vi "Item Selection Demo.vi"() -> ()   [LabVIEW 2020]
doc: "This is a Demo VI used to demonstrate how the listbox and tree selection VIs work. Run the VI and then select items by clicking the symbols of the controls. Use Shift to select multiple items, and right click the control to use other options.\n-------------\nBrian Hoover (hooovahh)"
uses:
  Selection Global Method.ctl
panel:
  out "Tree Selection":string[](array[string])
  in  "Tree":string(tree)
  out "MCLB Selection":string[](array[string])
  out "SCLB Selection":string[](array[string])
  in  "Multicolumn Listbox":i32(listbox)=-1
  in  "Listbox":i32(listbox)=-1
  # "1) Run This VI\n2) Click the checkboxes to select and unselect items.\n3) Shift can be held to change the selection of multiple items\n4) Right click the control to change the selection.\n5) Disabled items cannot be changed."
  # "Tree controls are supported with selection and deselection of parents affecting the children.  Deselecting and selecting children also will change the icon of the parent."
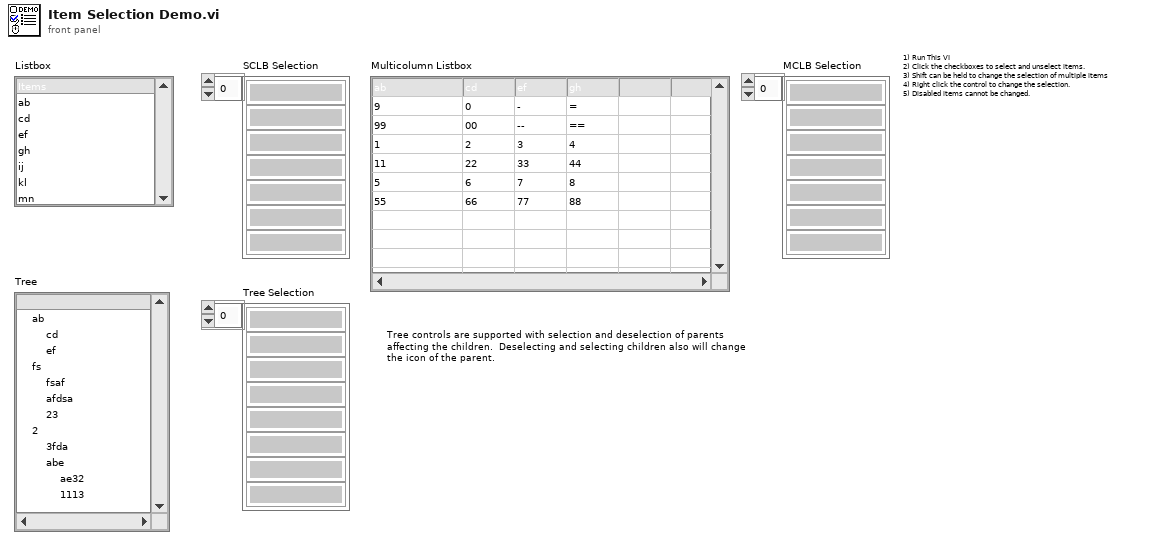
[diagram p1: front panel]
types:
  T1 = typedef "Selection Global Method.ctl" = enum16{"Read Selection", "Force Selection", "Mouse Down Event", "Select All", "Select None", "Invert Selection", "Read Selection and Tags"}
  T2 = typedef "LVPoint32TypeDef.ctl" = cluster{"Horizontal":i32, "Vertical":i32}
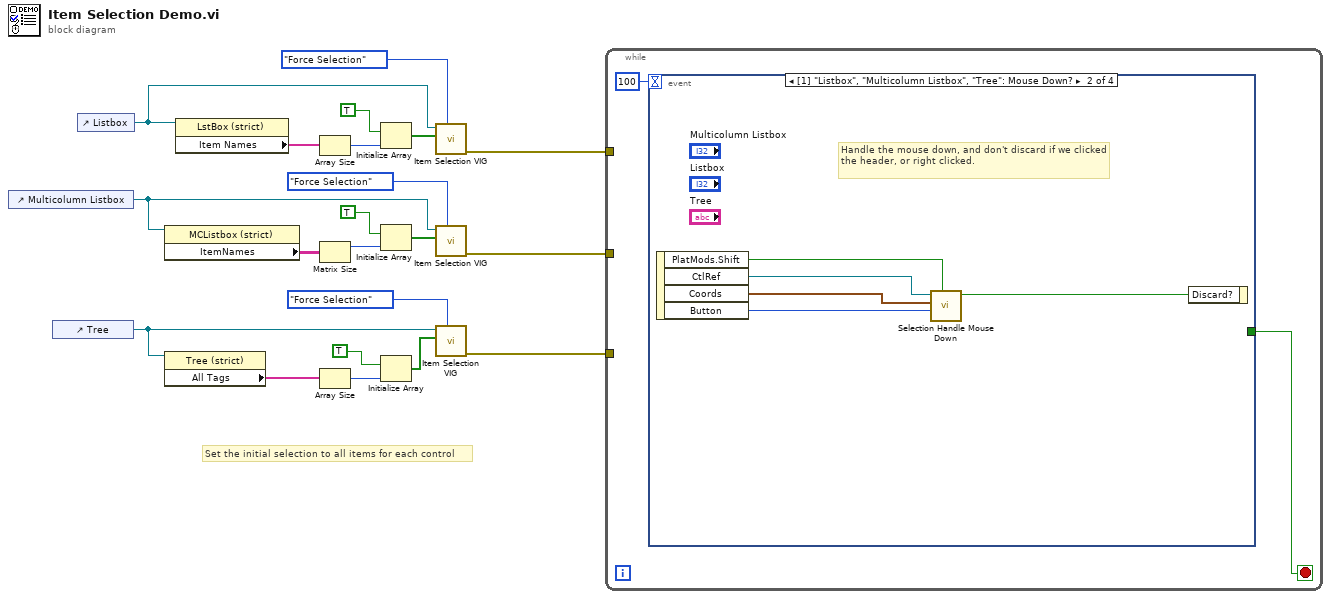
[diagram p0: block diagram]
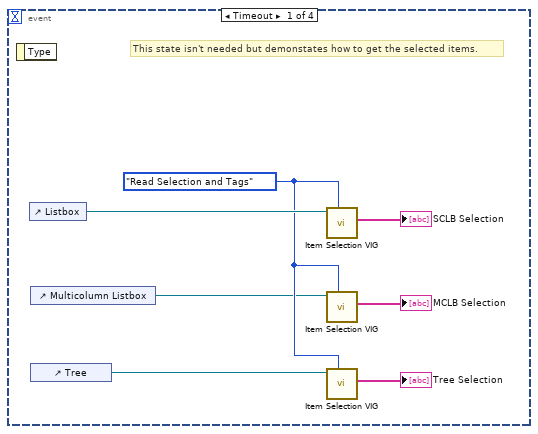
[diagram p2: hidden frame]
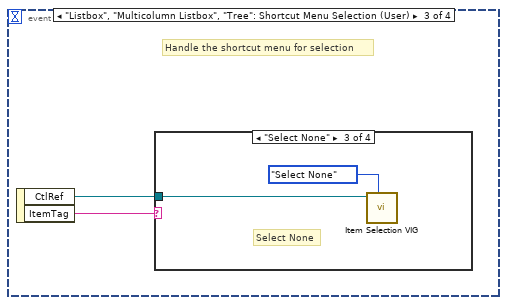
[diagram p3: hidden frame]
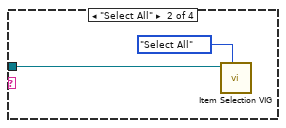
[diagram p5: hidden frame]
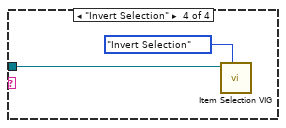
[diagram p6: hidden frame]
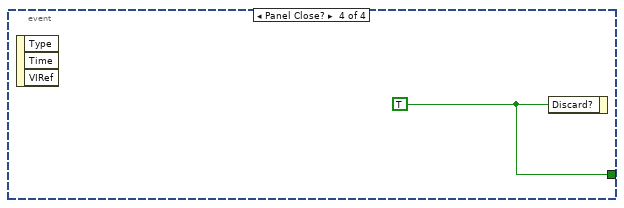
[diagram p7: hidden frame]
diagram:
  # "Set the initial selection to all items for each control"
  n1 = control-ref of="Multicolumn Listbox"() -> (w11:refnum<vi>)
  n2 = control-ref of="Tree"() -> (w2:refnum<vi>)
  n3 = control-ref of="Listbox"() -> (w6:refnum<vi>)
  n4 = property on="Property Node" class="MCListbox (strict)"(reference=w11) -> ("ItemNames"=w12:string[][])  [unwired: 1 in, 2 out]
  n5 = property class="Tree (strict)"(reference=w2) -> ("All Tags"=w1:string[])  [unwired: 1 in, 2 out]
  n6 = property on="Property Node" class="LstBox (strict)"(reference=w6) -> ("Item Names"=w10:string[])  [unwired: 1 in, 2 out]
  n7 = Array Size(array=w10) -> (size(s)=w9:i32)
  n8 = Matrix Size(0:w12) -> (1:w13:i32)  [unwired: 1 out]
  n9 = Array Size(array=w1) -> (size(s)=w18:i32)
  n10 = Initialize Array(TRUE, w9) -> (w7:bool[])
  n11 = Initialize Array(TRUE, w13) -> (w15:bool[])
  n12 = Initialize Array(TRUE, w18) -> (w16:bool[])
  n13 = call "Item Selection VIG.vi"("Method (Read Selection)"=Selection_Global_Method."Force Selection", "Selection"=w7, "Listbox or Tree"=w6) -> ("error out"=w21:errorcluster)  [unwired: 6 in, 2 out]
  n14 = call "Item Selection VIG.vi"("Method (Read Selection)"=Selection_Global_Method."Force Selection", "Selection"=w15, "Listbox or Tree"=w11) -> ("error out"=w20:errorcluster)  [unwired: 6 in, 2 out]
  n15 = call "Item Selection VIG.vi"("Method (Read Selection)"=Selection_Global_Method."Force Selection", "Selection"=w16, "Listbox or Tree"=w2) -> ("error out"=w3:errorcluster)  [unwired: 6 in, 2 out]
  n16 = while {
    tunnel: w21 -> [_]
    tunnel: w20 -> [_]
    tunnel: w3 -> [_]
    stop <- w23 stop-if-true
    n17 = event shown="[1] \"Listbox\", \"Multicolumn Listbox\", \"Tree\": Mouse Down?" {
      selector: _ -> [_ _ _ _]
      dyn-events: _ -> [_ _ _ _]
      timeout: 100 -> [_ _ _ _]
      tunnel: [_ _ _ w44] -> w23
      event Timeout {
        w26 = Selection_Global_Method."Read Selection and Tags" ("Method (Read Selection)")
        # "This state isn't needed but demonstates how to get the selected items."
        n18 = event-data() -> ()  [unwired: 1 in, 1 out]
        n19 = control-ref of="Listbox"() -> (w30:refnum<vi>)
        n20 = control-ref of="Multicolumn Listbox"() -> (w25:refnum<vi>)
        n21 = control-ref of="Tree"() -> (w29:refnum<vi>)
        n22 = call "Item Selection VIG.vi"("Method (Read Selection)"=w26, "Listbox or Tree"=w30) -> ("Tags"=→"SCLB Selection":string[])  [unwired: 7 in, 2 out]
        n23 = call "Item Selection VIG.vi"("Method (Read Selection)"=w26, "Listbox or Tree"=w25) -> ("Tags"=→"MCLB Selection":string[])  [unwired: 7 in, 2 out]
        n24 = call "Item Selection VIG.vi"("Method (Read Selection)"=w26, "Listbox or Tree"=w29) -> ("Tags"=→"Tree Selection":string[])  [unwired: 7 in, 2 out]
      }
      event "Listbox", "Multicolumn Listbox", "Tree": Mouse Down? {
        # "Handle the mouse down, and don't discard if we clicked the header, or right clicked."
        n25 = event-data() -> ("PlatMods.Shift"=w33:bool, "CtlRef"=w34:refnum<vi>, "Coords"=w32:T2, "Button"=w31:u16)  [unwired: 1 in]
        n26 = call "Selection Handle Mouse Down.vi"("Shift?"=w33, "Mouse Button"=w31, "Mouse Coords"=w32, "Listbox or Tree"=w34) -> ("Discard?"=w35:bool)  [unwired: 6 in, 1 out]
        n27 = event-data("Discard?"=w35) -> ()  [unwired: 1 in, 1 out]
      }
      event "Listbox", "Multicolumn Listbox", "Tree": Shortcut Menu Selection (User) {
        # "Handle the shortcut menu for selection"
        n28 = event-data() -> ("CtlRef"=w37:refnum<vi>, "ItemTag"=w36:string)  [unwired: 1 in]
        n29 = case shown="\"Select None\"" w36 {
          tunnel: w37 -> [_ w39 w41 w43]
          frame Default {
          }
          frame "Select All" {
            n30 = call "Item Selection VIG.vi"("Method (Read Selection)"=Selection_Global_Method."Select All", "Listbox or Tree"=w39) -> ()  [unwired: 7 in, 3 out]
          }
          frame "Select None" {
            # "Select None"
            n31 = call "Item Selection VIG.vi"("Method (Read Selection)"=Selection_Global_Method."Select None", "Listbox or Tree"=w41) -> ()  [unwired: 7 in, 3 out]
          }
          frame "Invert Selection" {
            n32 = call "Item Selection VIG.vi"("Method (Read Selection)"=Selection_Global_Method."Invert Selection", "Listbox or Tree"=w43) -> ()  [unwired: 7 in, 3 out]
          }
        }
      }
      event Panel Close? {
        w44 = TRUE ("Discard?")
        n33 = event-data() -> ()  [unwired: 1 in, 3 out]
        n34 = event-data("Discard?"=w44) -> ()  [unwired: 1 in, 1 out]
      }
    }
  }
